vi "test_pid_output_data_path.vi"() -> ()   [LabVIEW 2013]
panel:
  out "Waveform Graph 2":i16[](graph)
  out "Waveform Graph":dbl[][](graph)
  out "size(s)":i32
  in  "Fi_start":fxp<+/-,32,4>
  in  "Fi_delta":fxp<+/-,32,4>
  in  "Kd/Tau":fxp<+/-,32,4>
  in  "Kp":fxp<+/-,32,4>
  in  "Ki*Tau":fxp<+/-,32,4>
  in  "Enabled":bool=TRUE
  in  "AM phase":fxp<+,64,64>
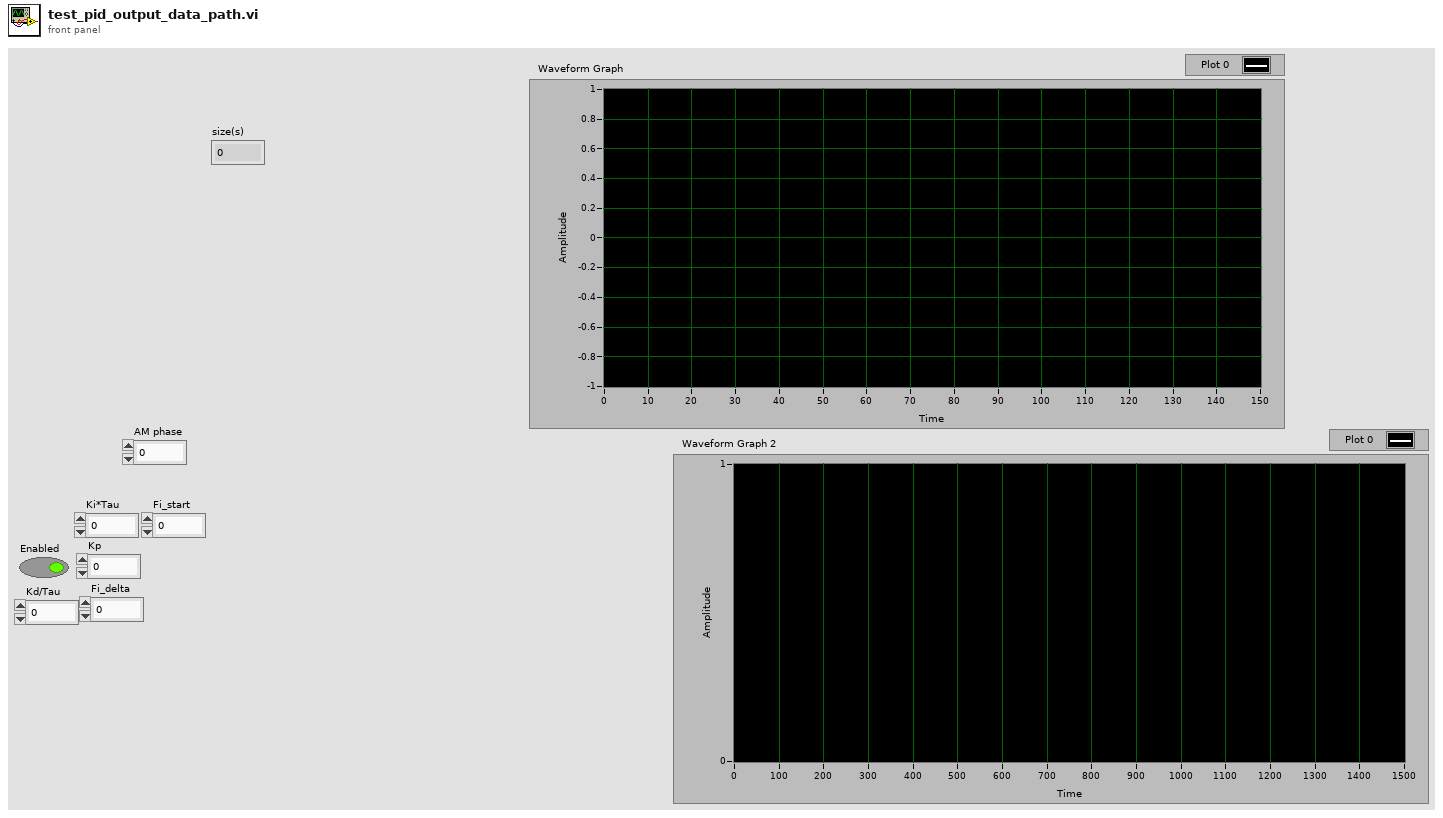
[diagram p1: front panel]
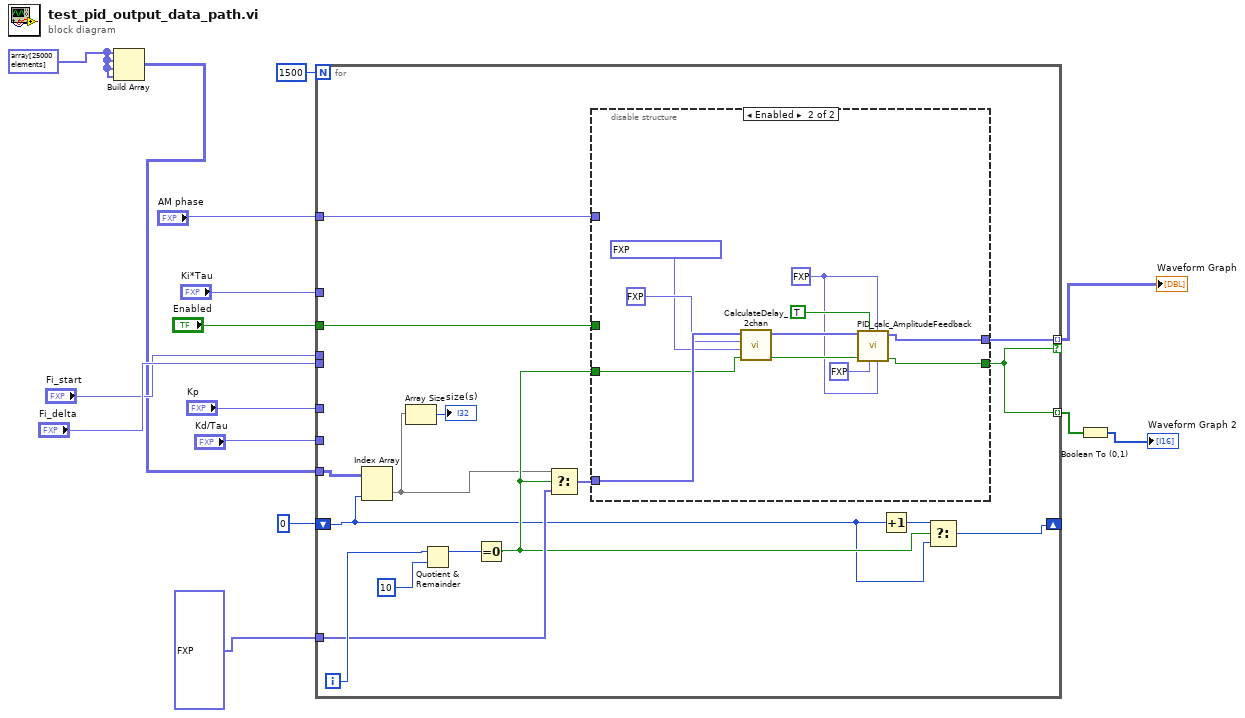
[diagram p0: block diagram]
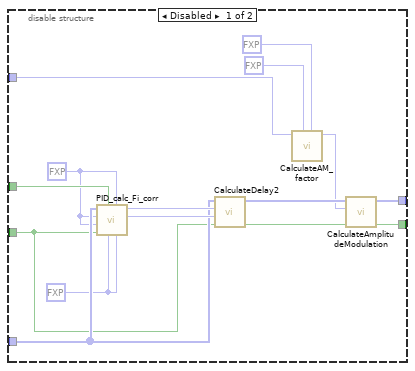
[diagram p2: hidden frame]
diagram:
  w7 = fxp<+/-,16,14>[] array[25000 elements] ("Array")
  n1 = Build Array(w7, w7, w7, w7) -> (w6:fxp<+/-,16,14>[][])
  n2 = for {
    N: 1500 -> [_]
    tunnel: "AM phase" -> [w31]
    tunnel: "Fi_delta" -> [_]
    tunnel: "Fi_start" -> [_]
    tunnel: "Enabled" -> [w30]
    tunnel: "Ki*Tau" -> [_]
    tunnel: "Kp" -> [_]
    tunnel: "Kd/Tau" -> [_]
    tunnel: fxp<+/-,16,14>[] [0.0, 0.0, 0.0, 0.0] ("Data in") -> [w26]
    tunnel: [w24] -> w1 mode=indexing if=w16
    tunnel: w6 -> [w23]
    shift-right: [w19] -> _
    shift-left: 0 ("y") -> [w20]
    tunnel: [w16] -> w3 mode=indexing
    i -> [w27]
    n3 = Index Array(array=w23, index (col)=w20) -> (element=w18:fxp<+/-,16,14>[])  [unwired: 1 in]
    n4 = Array Size(array=w18) -> (size(s)=→"size(s)":i32)
    n5 = Quotient & Remainder(x=w27, y=10) -> (x-y*floor(x/y)=w28:i32)  [unwired: 1 out]
    n6 = Equal To 0?(x=w28) -> (x = 0?=w21:bool)
    n7 = Select(t=w18, s=w21, f=w26) -> (s? t:f=w25:fxp<+/-,16,14>[])
    n8 = disable-structure shown="Enabled" {
      disable-tunnel: w31 -> [w41 _]
      disable-tunnel: w30 -> [w40 _]
      disable-tunnel: w25 -> [w37 w55]
      disable-tunnel: [w36 w48] -> w24
      disable-tunnel: w21 -> [w32 w52]
      disable-tunnel: [w33 w51] -> w16
      frame Disabled {
        w34 = fxp<+/-,32,4> 0.0 ("Kp")
        w35 = fxp<+/-,32,4> 0.0 ("Kp")
        n9 = call "PID_calc_Fi_corr.vi"("Kd/Tau"=w35, "Ki*Tau"=w34, "Kp"=w35, "Enabled"=w40, "input valid"=w32, "Fi_delta"=w34, "Fi_start"=w34, "Data in"=w37) -> ("cos_fi_korr"=w42:fxp<+/-,16,2>, "sin fi_korr"=w43:fxp<+/-,16,2>)  [unwired: 1 in, 1 out]
        n10 = call "CalculateDelay2.vi"("input valid"=w32, "cos_fi"=w42, "sin fi"=w43, "Data in"=w37) -> ("output valid"=w45:bool, "Data out"=w46:fxp<+/-,16,14>[])  [unwired: 6 in]
        n11 = call "CalculateAM_factor.vi"("b_am"=fxp<+/-,16,2> 0.0, "a_am"=fxp<+/-,16,2> 1.0, "AM phase"=w41) -> ("AM_factor"=w44:fxp<+/-,16,2>)  [unwired: 7 in, 1 out]
        n12 = call "CalculateAmplitudeModulation.vi"("input valid"=w45, "AM_factor"=w44, "Data in"=w46) -> ("output valid"=w33:bool, "Data out"=w36:fxp<+/-,16,14>[])  [unwired: 7 in]
      }
      frame Enabled {
        w49 = fxp<+/-,32,6> 0.0 ("Ki*Tau")
        n13 = call "CalculateDelay_2chan.vi"("input valid"=w52, "cos_fi"=fxp<+/-,16,0> 0.4999847412109375, "sin fi"=fxp<+/-,16,0> 0.0, "Data in"=w55) -> ("output valid"=w56:bool, "Data out"=w57:fxp<+/-,16,14>[])  [unwired: 6 in]
        n14 = call "PID_calc_AmplitudeFeedback.vi"("Kd/Tau"=w49, "Ki*Tau"=w49, "Kp"=fxp<+/-,32,6> 1.0, "Enabled"=TRUE, "input valid"=w56, "Data in"=w57) -> ("output valid"=w51:bool, "data out"=w48:fxp<+/-,16,14>[])  [unwired: 2 in, 2 out]
      }
    }
    n15 = Increment(x=w20) -> (x+1=w22:i32)
    n16 = Select(t=w22, s=w21, f=w20) -> (s? t:f=w19:i32)
  }
  "Waveform Graph" <- w1
  n17 = Boolean To (0,1)(Boolean=w3) -> (0, 1=→"Waveform Graph 2":i16[])
